vi "IMU and RoboteQ.vi"() -> ()   [LabVIEW 2012]
uses:
  MicroStrain/LabVIEW Library v2/AHRS/Controls/Desciptor Set Byte.ctl
  <vilib>/robotics/Controls/Attitude Indicator/Attitude Indicator.xctl
  <vilib>/Platform/TimedLoop/XDataNode/timing_clust.ctl
  <vilib>/Platform/TimedLoop/XDataNode/nitl_modes.ctl
  <vilib>/Platform/TimedLoop/XDataNode/wakeup.ctl
  Labview/Public/Set Control Effort.vi
  <vilib>/Instr/_visa.llb/VISA Configure Serial Port (Instr).vi
  MicroStrain/LabVIEW Library v2/AHRS/SubVI/3DM-GX3-45 Commands/Start Stream.vi
  MicroStrain/LabVIEW Library v2/AHRS/SubVI/3DM-GX3-45 Commands/Stop Stream.vi
  <vilib>/Platform/TimedLoop/XDataNode/XDataNode.xnode
  Labview/Roboteq.lvlib
  <vilib>/Platform/TimedLoop/XDataNode/XDNodeRunTimeDep.lvlib
panel:
  in  "IMU VISA":refnum<visa-resource-name>="COM5"
  out "Error Out":errorcluster
  in  "Error In":errorcluster
  out "Received Array":u8[](array[numeric]) format="%02x"
  out "Processing Loop Count":i32
  out "Received array Size":i32
  out "Attitude Indicator":cluster{"Roll":dbl, "Pitch":dbl}(xcontrol)
  out "YAW":dbl(knob) scale=-180.0..180.0
  out "result string":string
  out "Read Loop Count":i32
  in  "Stop Data Stream":bool
  in  "Start Data Stream":bool
  in  "Self Test":bool
  out "Serial Settings:Number of Bytes at Serial Port":u32
  out "timed out?":bool
  in  "Field Data":u8[](array[numeric]) format="%02x"
  in  "Field Descriptor Byte":u8=117 format="%02x"
  in  "Data Set":T1=enum."NAV"
  in  "ID Query (True)":bool
  in  "Motor1 Effort":i32(slide) scale=-10.0..10.0
  in  "Motor2 Effort":i32(slide) scale=-10.0..10.0
  in  "End Loop":bool
  in  "stop?":bool
  out "Telemetry":T2={"Voltage"={0.0, 0.0, 0.0}, "Encoder Speed"={0, 0}, "Temps"={"IC Temp (C)"=0, "Ch1 Temp (C)"=0, "Ch2 Temp (C)"=0}, "Current"={0.0, 0.0, 0.0, 4.6238981750249924e+36}} {"Current" scale=0.0..16.0; "Temps"."IC Temp (C)" scale=0.0..150.0; "Temps"."Ch1 Temp (C)" scale=0.0..150.0; "Temps"."Ch2 Temp (C)" scale=0.0..150.0; "Encoder Speed" scale=-100.0..100.0; "Voltage" scale=8.0..14.0}
  out "Command to Serial":string
  in  "RoboteQ VISA":refnum<visa-resource-name>
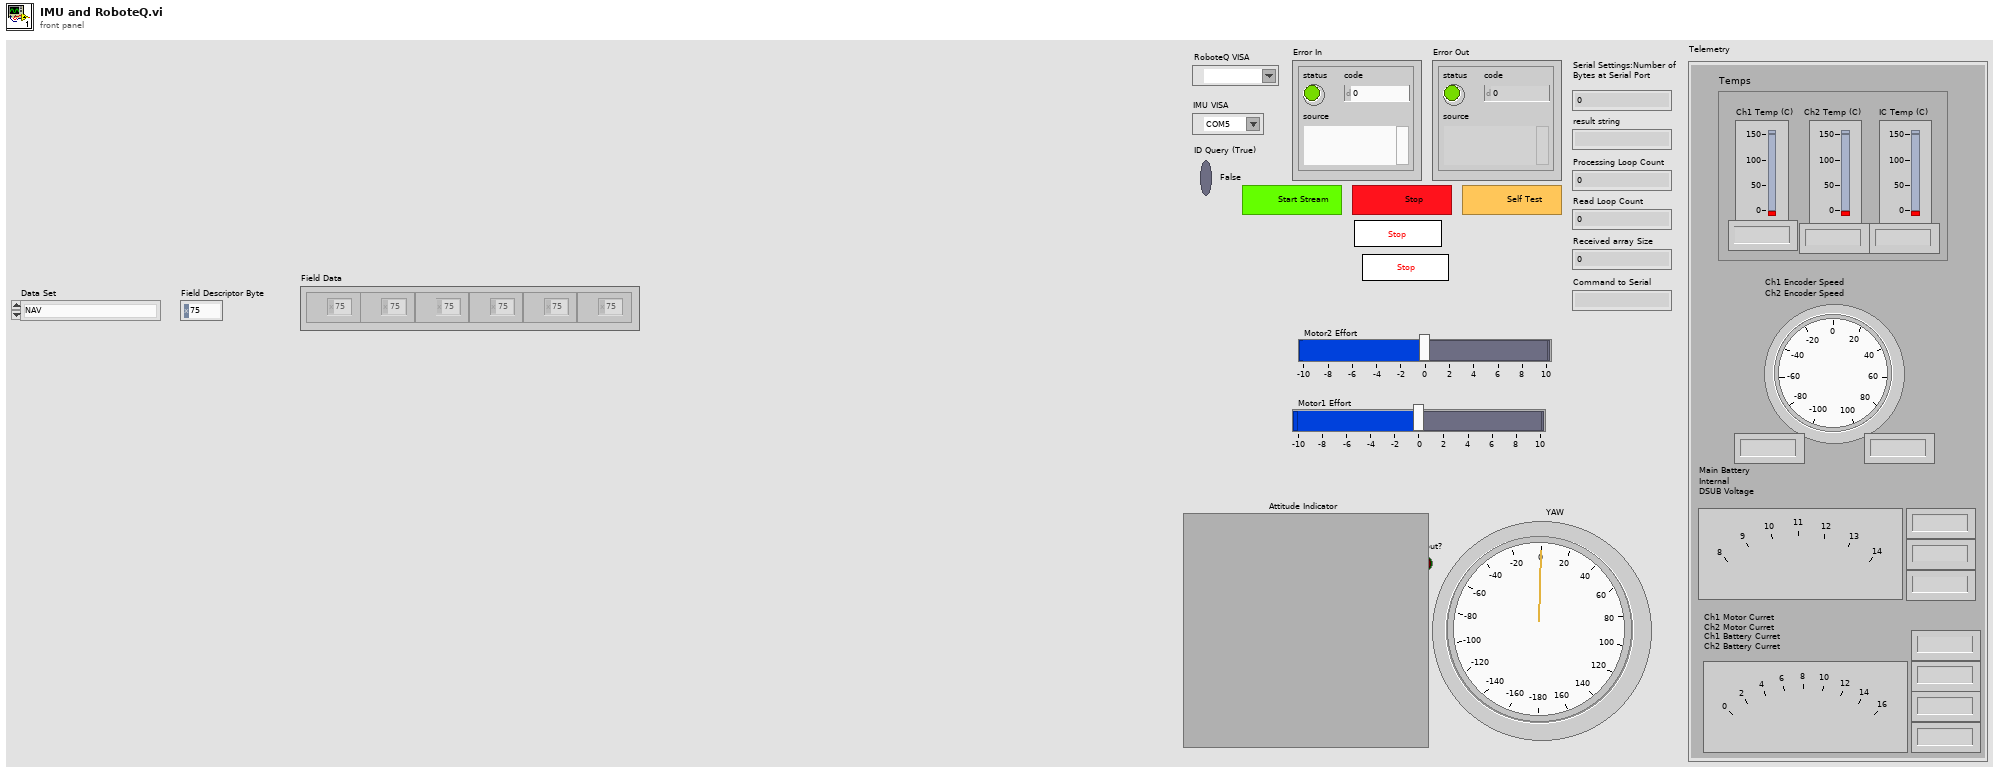
[diagram p1: front panel]
types:
  T1 = typedef "Desciptor Set Byte.ctl" = enum16{"Base Command Set", "3DM Command Set", "Navigation Filter Command Set", "System Command Set", "AHRS", "GPS", "NAV"}
  T2 = cluster{"Voltage":cluster{sgl, sgl, sgl}, "Encoder Speed":cluster{i32, i32}, "Temps":cluster{"IC Temp (C)":i32, "Ch1 Temp (C)":i32, "Ch2 Temp (C)":i32}, "Current":cluster{dbl, dbl, dbl, dbl}}
  T3 = typedef "XDNodeRunTimeDep.lvlib/timing_clust.ctl" = cluster{"Expected End [f-1]":u64, "Actual End [f-1]":u64, "Finished Late? [f-1]":bool, "Expected End [i-1]":u64, "Actual End [i-1]":u64, "Finished Late? [i-1]":bool, "Expected Start [i]":u64, "Actual Start [i]":u64, "Expected Start [f]":u64, "Actual Start [f]":u64, "Source Name":string, "Structure Name":string, "Period":i64, "Deadline":i64, "Offset":i64, "Start":i64, "Priority":i32, "Timeout":i32, "Mode":T4, "Wakeup Reason":T5, "Error":errorcluster, "Source Type":string, "Secondary Source Type":string, "Global End Time":u64, "Global Start Time":u64, "Frame Duration":u64, "Iteration Duration":u64, "Assigned CPU":i32, "I/O Scan Engine Mode":u32}
  T4 = typedef "XDNodeRunTimeDep.lvlib/nitl_modes.ctl" = enum32{"No Change", "Process missed periods, maintain original phase", "Discard missed periods, maintain original phase", "Process missed periods, ignore original phase", "Discard missed periods, ignore original phase"}
  T5 = typedef "XDNodeRunTimeDep.lvlib/wakeup.ctl" = enum32{"Normal", "Aborted", "Asynchronous wakeup", "Timing source error", "Timed loop error", "Timeout"}
  T6 = cluster{"main battery voltage (V)":sgl, "internal voltage (V)":sgl, "DSUB voltage (V)":sgl}
  T7 = cluster{" Ch1  Motor current (I)":sgl, " Ch2 Motor current (I)":sgl, " Ch1 Battery current (I)":sgl, " Ch2 Battery current (I)":sgl}
  T8 = cluster{"Ch1 Temp (C)":i32, "Ch2 Temp (C)":i32, "IC Temp (C)":i32}
  T9 = cluster{"Encoder Speed (RPM)":i32, "Encoder Speed (RPM)":i32}
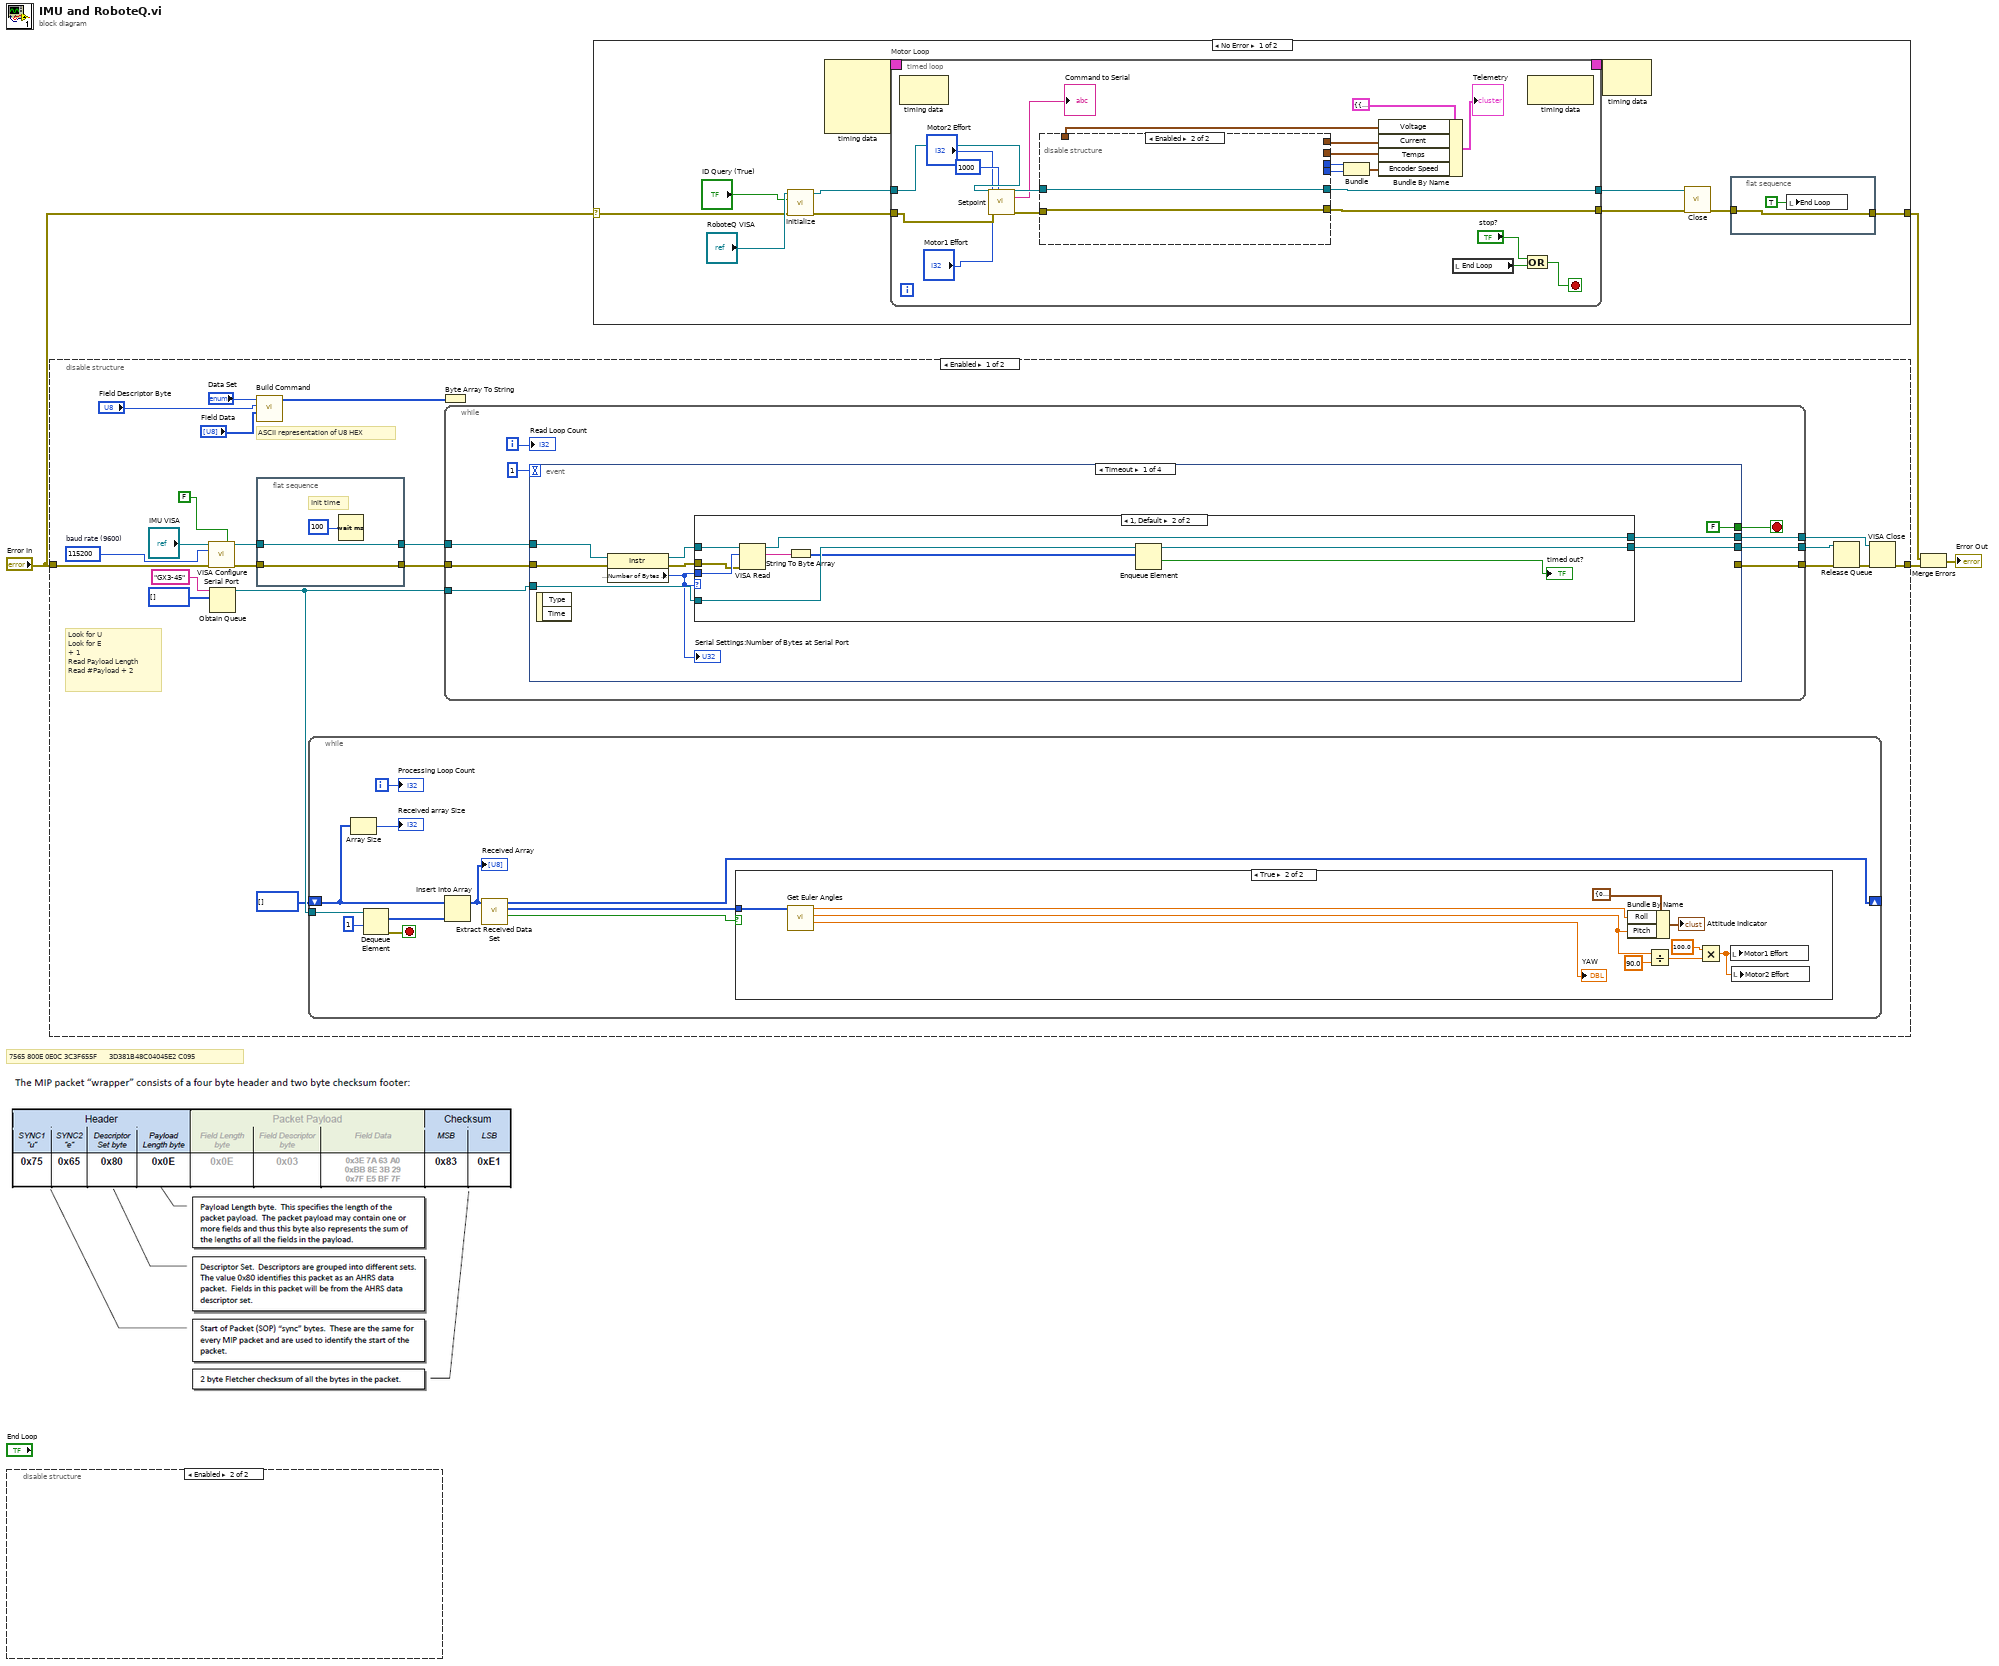
[diagram p0: block diagram]
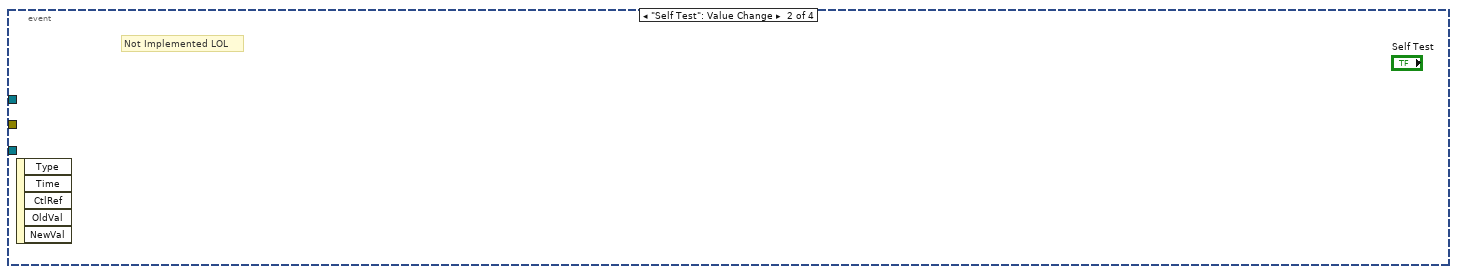
[diagram p4: hidden frame]
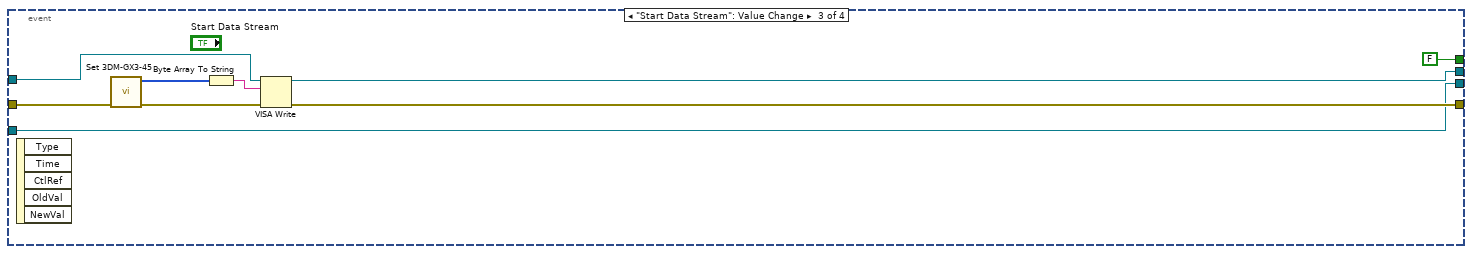
[diagram p5: hidden frame]
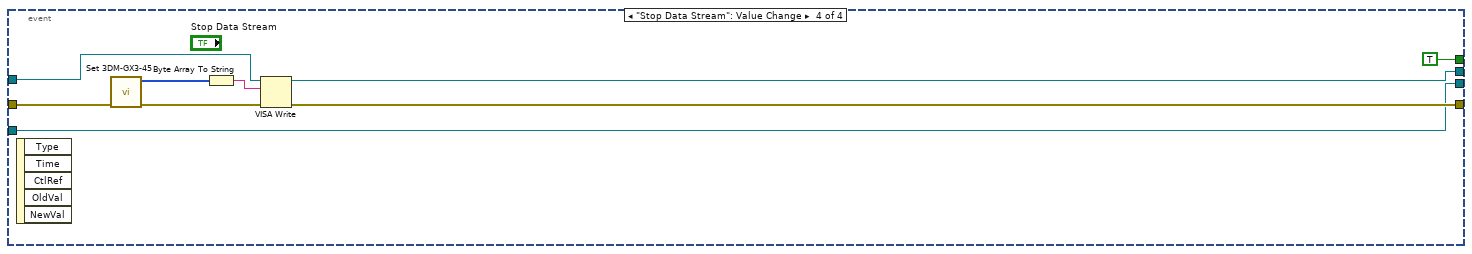
[diagram p6: hidden frame]
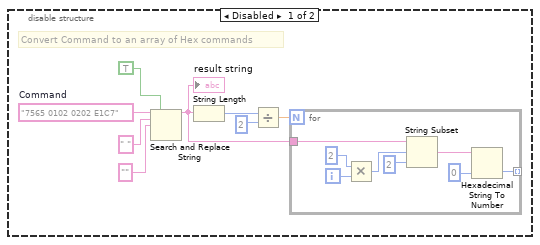
[diagram p8: hidden frame]
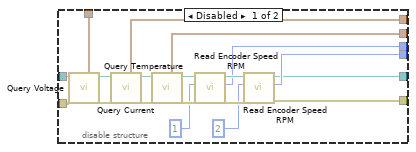
[diagram p9: hidden frame]
diagram:
  # "7565 800E 0E0C 3C3F655F      3D381B48C04045E2 C095"
  n1 = disable-structure shown="Enabled" {
    frame Disabled {
      w12 = "7565 0102 0202 E1C7"  # Command
      # "Convert Command to an array of Hex commands"
      n2 = Search and Replace String(replace all?=TRUE ("replace all? (F)"), input string=w12, search string=" ", replace string="" ("replace string (\"\")")) -> (result string=w8:string)  [unwired: 4 in, 3 out]
      "result string" <- w8
      n3 = String Length(string=w8) -> (length=w7:i32)
      n4 = Divide(x=w7, y=2) -> (x/y=w5:dbl)
      n5 = for {
        N: w5 -> [_]
        tunnel: w8 -> [w20]
        tunnel: [w13] -> _ mode=indexing
        i -> [w18]
        n6 = Multiply(x=2, y=w18) -> (x*y=w16:i32)
        n7 = String Subset(string=w20, offset (0)=w16, length (rest)=2 ("length (rest)")) -> (substring=w15:string)
        n8 = Hexadecimal String To Number(string=w15, default (0uL)=u8 0 ("default (0 U32)")) -> (number=w13:u8)  [unwired: 1 in, 1 out]
      }
    }
    frame Enabled {
    }
  }
  n9 = disable-structure shown="Enabled" {
    disable-tunnel: [w22 w113] -> w2
    disable-tunnel: "Error In" -> [w21 w113]
    frame Enabled {
      w37 = u32 115200  # baud rate (9600)
      # "Look for U\nLook for E\n+ 1\nRead Payload Length\nRead #Payload + 2"
      # "ASCII representation of U8 HEX"
      n10 = call-poly "VISA Configure Serial Port"("VISA resource name"="IMU VISA", "Enable Termination\nChar (T)"=FALSE ("Enable Termination\nChar (T)"), "baud rate (9600)"=w37, "error in (no error)"=w21) -> ("VISA resource name out"=w27:refnum<visa-resource-name>, "error out"=w24:errorcluster)  [unwired: 10 in]
      n11 = Obtain Queue(name (unnamed)="GX3-45", element data type=u8[] [] ("unsigned byte array")) -> (queue out=w30:refnum<queue>)  [unwired: 3 in, 2 out]
      n12 = call "Build Command.vi"("Field Data"="Field Data", "Field Descriptor Byte"="Field Descriptor Byte", "Data Set"="Data Set") -> ("Command"=w33:u8[])  [unwired: 7 in, 1 out]
      n13 = flat-sequence {
        tunnel: w27 -> [w112]
        tunnel: [w112] -> w36
        tunnel: w24 -> [w110]
        tunnel: [w110] -> w23
        frame #0 {
          # "Init time"
          n14 = Wait (ms)(milliseconds to wait=u32 100) -> ()  [unwired: 1 out]
        }
      }
      n15 = while {
        tunnel: w30 -> [w52]
        shift-right: [w46] -> _
        shift-left: u8[] [] ("element") -> [w44]
        i -> [w49]
        stop <- w51 stop-if-true
        n16 = Array Size(array=w44) -> (size(s)=→"Received array Size":i32)
        n17 = Dequeue Element(queue=w52, timeout in ms (-1)=1) -> (element=w50:u8[], error out=w51:errorcluster)  [unwired: 1 in, 2 out]
        n18 = Insert Into Array(array=w44, new element=w50) -> (w48:u8[])  [unwired: 1 in]
        "Received Array" <- w48
        n19 = call "Extract Received Data Set.vi"("Received Array In"=w48) -> ("New Data Set Received"=w43:bool, "Extracted Data Set"=w47:u8[], "Received Array Out"=w46:u8[])  [unwired: 7 in, 1 out]
        n20 = case shown="True" w43 {
          tunnel: w47 -> [_ w62]
          frame False {
          }
          frame True {
            n21 = call "Get Euler Angles.vi"("Received Array"=w62) -> ("Yaw (deg)"=→"YAW":dbl, "Pitch (deg)"=w54:dbl, "Roll (deg)"=w58:dbl)  [unwired: 7 in]
            n22 = Bundle By Name(cluster=cluster{"Roll":dbl, "Pitch":dbl} {"Roll"=0.0, "Pitch"=0.0} ("Attitude Indicator 2"), "Roll"=w58, "Pitch"=w54) -> (→"Attitude Indicator":cluster{"Roll":dbl, "Pitch":dbl})
            n23 = Divide(x=w54, y=90.0) -> (x/y=w56:dbl)
            n24 = Multiply(x=100.0, y=w56) -> (x*y=w53:dbl)
            n25 = local write "Motor1 Effort"(w53) -> ()
            n26 = local write "Motor2 Effort"(w53) -> ()
          }
        }
        "Processing Loop Count" <- w49
      }
      n27 = Byte Array To String(unsigned byte array=w33) -> ()  [unwired: 1 out]
      n28 = while {
        tunnel: w36 -> [w71]
        tunnel: [w70] -> w34
        tunnel: w30 -> [w68]
        tunnel: [w67] -> w29
        tunnel: w23 -> [w65]
        tunnel: [w64] -> w26
        i -> [w69]
        stop <- w63 stop-if-true
        n29 = event shown="[0] Timeout" {
          selector: _ -> [_ _ _ _]
          dyn-events: _ -> [_ _ _ _]
          timeout: 1 -> [_ _ _ _]
          tunnel: w71 -> [w80 _ w100 w109]
          tunnel: [w78 _ w97 w106] -> w70
          tunnel: w68 -> [w76 _ w92 w101]
          tunnel: [w74 _ w92 w101] -> w67
          tunnel: w65 -> [w73 _ w96 w105]
          tunnel: [_ _ w94 w103] -> w64
          tunnel: [FALSE ("Stop Data Stream 2") _ FALSE ("Stop Data Stream 2") TRUE ("Stop Data Stream 2")] -> w63
          event Timeout {
            n30 = event-data() -> ()  [unwired: 1 in, 2 out]
            n31 = property class="Instr"(reference=w80, error in=w73) -> (reference out=w79:refnum<visa-resource-name>, error out=w77:errorcluster, "Serial Settings:Number of Bytes at Serial Port"=w75:u32)
            "Serial Settings:Number of Bytes at Serial Port" <- w75
            n32 = case shown="1, Default" w75 {
              tunnel: w79 -> [w82 w91]
              tunnel: [w82 w90] -> w78
              tunnel: w75 -> [_ w89]
              tunnel: w77 -> [_ w88]
              tunnel: w76 -> [w81 w86]
              tunnel: [w81 w83] -> w74
              frame 0 {
              }
              frame 1, Default {
                n33 = VISA Read(VISA resource name=w91, byte count=w89, error in (no error)=w88) -> (VISA resource name out=w90:refnum<visa-resource-name>, read buffer=w87:string)  [unwired: 2 out]
                n34 = String To Byte Array(string=w87) -> (unsigned byte array=w85:u8[])
                n35 = Enqueue Element(queue=w86, element=w85) -> (queue out=w83:refnum<queue>, timed out?=→"timed out?":bool)  [unwired: 2 in, 1 out]
              }
            }
          }
          event "Self Test": Value Change {
            # "Not Implemented LOL"
            n36 = event-data() -> ()  [unwired: 1 in, 5 out]
          }
          event "Start Data Stream": Value Change {
            n37 = event-data() -> ()  [unwired: 1 in, 5 out]
            n38 = call-poly "Set 3DM-GX3-45.vi"("Error In"=w96) -> ("Error Out"=w95:errorcluster, "Command"=w99:u8[])  [unwired: 9 in]
            n39 = Byte Array To String(unsigned byte array=w99) -> (string=w98:string)
            n40 = VISA Write(VISA resource name=w100, write buffer=w98, error in (no error)=w95) -> (VISA resource name out=w97:refnum<visa-resource-name>, error out=w94:errorcluster)  [unwired: 1 out]
          }
          event "Stop Data Stream": Value Change {
            n41 = event-data() -> ()  [unwired: 1 in, 5 out]
            n42 = call-poly "Set 3DM-GX3-45.vi"("Error In"=w105) -> ("Error Out"=w104:errorcluster, "Command"=w108:u8[])  [unwired: 9 in]
            n43 = Byte Array To String(unsigned byte array=w108) -> (string=w107:string)
            n44 = VISA Write(VISA resource name=w109, write buffer=w107, error in (no error)=w104) -> (VISA resource name out=w106:refnum<visa-resource-name>, error out=w103:errorcluster)  [unwired: 1 out]
          }
        }
        "Read Loop Count" <- w69
      }
      n45 = Release Queue(queue=w29, error in (no error)=w26) -> (error out=w25:errorcluster)  [unwired: 1 in, 2 out]
      n46 = VISA Close(VISA resource name=w34, error in (no error)=w25) -> (error out=w22:errorcluster)
    }
    frame Disabled {
    }
  }
  n47 = case shown="No Error" "Error In" {
    selector: "Error In" -> [w116 w173]
    tunnel: [w114 w173] -> w3
    frame No Error {
      n48 = call "Initialize.vi"("error in (no error)"=w116, "ID Query (True)"="ID Query (True)", "VISA resource name"="RoboteQ VISA") -> ("error out"=w121:errorcluster, "VISA resource name out"=w122:refnum<visa-resource-name>)  [unwired: 7 in]
      n49 = node-c288() -> (w118:T3)  [unwired: 4 in]
      n50 = timed-loop "Motor Loop" {
        tunnel: w122 -> [w143]
        tunnel: w121 -> [w142]
        tunnel: [w125] -> w120
        tunnel: [w138] -> w124
        timing: w118 -> [_]
        timing-out: [_] -> w117
        stop <- w144 stop-if-true
        n51 = node-c288() -> ()  [unwired: 1 in, 1 out]
        n52 = call-poly "Setpoint.vi"("Max Effort"=1000, "error in (no error)"=w142, "Motor2 Effort"="Motor2 Effort", "Motor1 Effort"="Motor1 Effort", "VISA resource name"=w143) -> ("error out"=w139:errorcluster, "Command"=→"Command to Serial":string, "VISA resource name out"=w140:refnum<visa-resource-name>)  [unwired: 4 in]
        n53 = disable-structure shown="Enabled" {
          disable-tunnel: w140 -> [w164 w166]
          disable-tunnel: w139 -> [w163 w165]
          disable-tunnel: [w158 _] -> w132
          disable-tunnel: [w157 _] -> w131
          disable-tunnel: [w147 w166] -> w138
          disable-tunnel: [w156 _] -> w133
          disable-tunnel: [w146 w165] -> w125
          disable-tunnel: [w155 _] -> w134
          disable-tunnel: [w150 _] -> w129
          frame Disabled {
            n54 = call "Query Voltage.vi"("error in (no error)"=w163, "VISA resource name"=w164) -> ("error out"=w153:errorcluster, "VISA resource name out"=w154:refnum<visa-resource-name>, "Voltages"=w155:T6)  [unwired: 4 in, 3 out]
            n55 = call "Query Current.vi"("error in (no error)"=w153, "VISA resource name"=w154) -> ("error out"=w151:errorcluster, "VISA resource name out"=w152:refnum<visa-resource-name>, "Motor Currents"=w150:T7)  [unwired: 3 in, 4 out]
            n56 = call "Query Temperature.vi"("error in (no error)"=w151, "VISA resource name"=w152) -> ("error out"=w161:errorcluster, "VISA resource name out"=w162:refnum<visa-resource-name>, "Temps"=w156:T8)  [unwired: 4 in, 3 out]
            n57 = call "Read Encoder Speed RPM.vi"("error in (no error)"=w161, "channel number"=u8 1, "VISA resource name"=w162) -> ("error out"=w159:errorcluster, "Encoder Speed (RPM)"=w158:i32, "VISA resource name out"=w160:refnum<visa-resource-name>)  [unwired: 6 in]
            n58 = call "Read Encoder Speed RPM.vi"("error in (no error)"=w159, "channel number"=u8 2, "VISA resource name"=w160) -> ("error out"=w146:errorcluster, "Encoder Speed (RPM)"=w157:i32, "VISA resource name out"=w147:refnum<visa-resource-name>)  [unwired: 6 in]
          }
          frame Enabled {
          }
        }
        n59 = Bundle("Encoder Speed (RPM)"=w132, "Encoder Speed (RPM)"=w131) -> (w130:T9)  [unwired: 1 in]
        n60 = Bundle By Name(cluster=T2 {"Voltage"={0.0, 0.0, 0.0}, "Encoder Speed"={0, 0}, "Temps"={"IC Temp (C)"=0, "Ch1 Temp (C)"=0, "Ch2 Temp (C)"=0}, "Current"={0.0, 0.0, 0.0, 0.0}} ("Telemetry"), "Voltage"=w134, "Current"=w129, "Temps"=w133, "Encoder Speed"=w130) -> (→"Telemetry":T2)
        n61 = local read "End Loop"() -> (w141:bool)
        n62 = node-c288() -> ()  [unwired: 1 in, 1 out]
        n63 = Compound Arithmetic op=OR("stop?", w141) -> (w144:bool)
      }
      n64 = node-c288(w117) -> ()  [unwired: 1 out]
      n65 = call "Close.vi"("error in (no error)"=w120, "VISA resource name"=w124) -> ("error out"=w119:errorcluster)  [unwired: 9 in]
      n66 = flat-sequence {
        tunnel: w119 -> [w171]
        tunnel: [w171] -> w114
        frame #0 {
          n67 = local write "End Loop"(TRUE ("End Loop")) -> ()
        }
      }
    }
    frame Error {
    }
  }
  n68 = Merge Errors(w3, w2) -> (→"Error Out":errorcluster)
